vi "Init HTTP.vi"(8 "error in (no error)":errorcluster, 11 "GodotServer in":refnum<class "GodotServer.lvclass">) -> (0 "error out":errorcluster, 3 "GodotServer out":refnum<class "GodotServer.lvclass">)   [LabVIEW 2020, in "GodotLV.lvlib" / "GodotServer.lvclass"]
uses:
  GodotServer.lvclass
  GodotServer.lvclass/GodotServer.ctl
  <vilib>/IlluminatedG/IG HTTP Server/HTTP Server/StandardFileServe/StandardFileServe.lvclass
  C:/Program Files (x86)/National Instruments/LabVIEW 2020/vi.lib/IlluminatedG/IG HTTP Server/HTTP Server/Handler/Handler.lvclass
  GodotHeaders/GodotHeaders.lvclass
  <vilib>/IlluminatedG/IG HTTP Server/HTTP Server/Server/Add Connection Handler.vi
  <vilib>/IlluminatedG/IG HTTP Server/HTTP Server/Server/Add Request Handler.vi
  <vilib>/IlluminatedG/IG HTTP Server/HTTP Server/Server/Add Route Handler.vi
  <vilib>/IlluminatedG/IG HTTP Server/HTTP Server/Server/Add Controller Handler.vi
  <vilib>/IlluminatedG/IG HTTP Server/HTTP Server/Server/Add Controller.vi
  <vilib>/IlluminatedG/IG HTTP Server/HTTP Server/Server/Add Response Handler.vi
  <vilib>/IlluminatedG/IG HTTP Server/HTTP Server/Server/Add Complete Handler.vi
  <vilib>/IlluminatedG/IG HTTP Server/HTTP Server/Server/Add Exception Handler.vi
  WebSocket Connection State Callback.vi
  <vilib>/IlluminatedG/IG HTTP Server/HTTP Server/Connection Handler/Connection Handler.lvclass
  <vilib>/IlluminatedG/IG HTTP Server/HTTP Server/Request Handler/Request Handler.lvclass
  <vilib>/IlluminatedG/IG HTTP Server/HTTP Server/Route Handler/Route Handler.lvclass
  <vilib>/IlluminatedG/IG HTTP Server/HTTP Server/Controller Handler/Controller Handler.lvclass
  <vilib>/IlluminatedG/IG HTTP Server/HTTP Server/Controller/Controller.lvclass
  <vilib>/IlluminatedG/IG HTTP Server/HTTP Server/Response Handler/Response Handler.lvclass
  <vilib>/IlluminatedG/IG HTTP Server/HTTP Server/Complete Handler/Complete Handler.lvclass
  <vilib>/IlluminatedG/IG HTTP Server/HTTP Server/Exception Handler/Exception Handler.lvclass
  <vilib>/IlluminatedG/IG HTTP Server/HTTP Server/Handler/Handler.lvclass
  <vilib>/IlluminatedG/IG WebSocket Stream/Stream-Websocket/Websocket Server/Websocket Server.lvclass
  <vilib>/IlluminatedG/IG HTTP Server/HTTP Server/Server/Server.lvclass
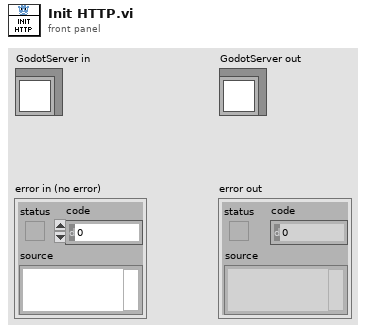
[diagram p1: front panel]
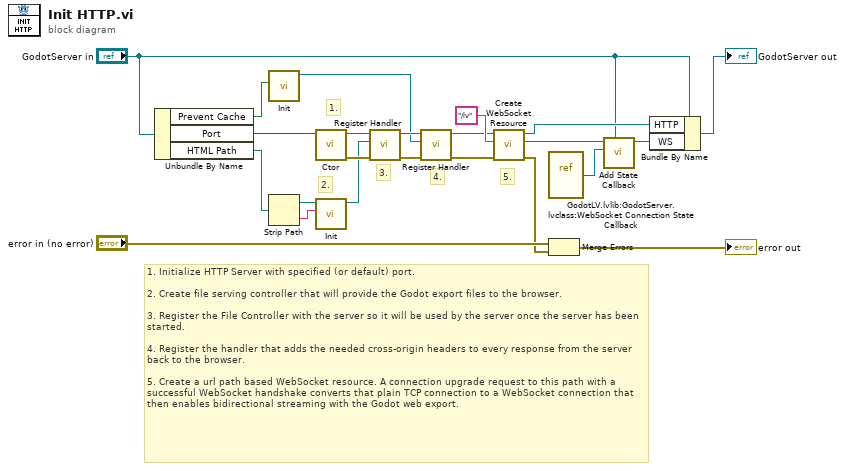
[diagram p0: block diagram]
diagram:
  # "1. Initialize HTTP Server with specified (or default) port.\n\n2. Create file serving controller that will provide the Godot export files to the browser.\n\n3. Register the File Controller with the server so it will be used by the server once the server has been started.\n\n4. Register the handler that adds the needed cross-origin headers to every response from the server back to the browser.\n\n5. Create a url path based WebSocket resource. A connection upgrade request to this path with a successful WebSocket handshake converts that plain TCP connection to a WebSocket connection that then enables bidirectional streaming with the Godot web export."
  # "5."
  # "4."
  # "3."
  # "2."
  # "1."
  n1 = Unbundle By Name("GodotServer in") -> ("Prevent Cache"=w2:bool, "Port"=w14:u16, "HTML Path"=w13:path)
  n2 = call <vilib>:"Init.vi"("Prevent Cache"=w2) -> ("GodotHeaders out"=w1:refnum<class "GodotHeaders.lvclass">)  [unwired: 9 in, 1 out]
  n3 = Strip Path(path=w13) -> (stripped path=w12:path, name=w11:string)
  n4 = call <vilib>:"Ctor.vi"("HTTP Port (80)"=w14) -> ("error out"=w22:errorcluster, "Server out"=w21:refnum<class "Server.lvclass">)  [unwired: 9 in]
  n5 = call <vilib>:"Init.vi"("Default Index File (index.html)"=w11, "Public Root"=w12) -> ("StandardFileServe out"=w20:refnum<class "StandardFileServe.lvclass">)  [unwired: 8 in, 1 out]
  n6 = call <vilib>:"Register Handler.vi"("error in (no error)"=w22, "Handler"=w20, "Server in"=w21) -> ("error out"=w16:errorcluster, "Server out"=w15:refnum<class "Server.lvclass">)  [unwired: 7 in]
  n7 = call <vilib>:"Register Handler.vi"("error in (no error)"=w16, "Handler"=w1, "Server in"=w15) -> ("error out"=w17:errorcluster, "Server out"=w18:refnum<class "Server.lvclass">)  [unwired: 7 in]
  n8 = call <vilib>:"Create WebSocket Resource.vi"("error in (no error)"=w17, "Path"="/lv", "Server in"=w18) -> ("error out"=w7:errorcluster, "WS Server"=w6:refnum<class "Websocket Server.lvclass">, "Server out"=w9:refnum<class "Server.lvclass">)  [unwired: 6 in]
  n9 = vi-ref "GodotLV.lvlib:GodotServer.lvclass:WebSocket Connection State Callback.vi"() -> (w3:refnum<vi>)
  n10 = Merge Errors("error in (no error)", w7) -> (→"error out":errorcluster)
  n11 = call-dynamic "Add State Callback.vi"("Owner (None)"="GodotServer in", "Callback"=w3, "Endpoint in"=w6) -> ("Endpoint out"=w5:refnum<class "Websocket Server.lvclass">)  [unwired: 7 in, 1 out]
  n12 = Bundle By Name(cluster="GodotServer in", "HTTP"=w9, "WS"=w5) -> (→"GodotServer out":refnum<class "GodotServer.lvclass">)
